vi "InsertReportSection.vi"(8 "error in (no error)":errorcluster, 10 "report entry":string, 11 "report section in":refnum<k7>) -> (0 "error out":errorcluster, 3 "report section out":refnum<k7>)   [LabVIEW 2019]
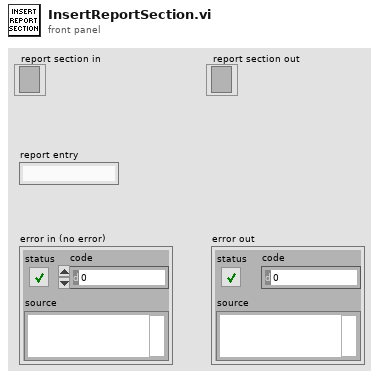
[diagram p1: front panel]
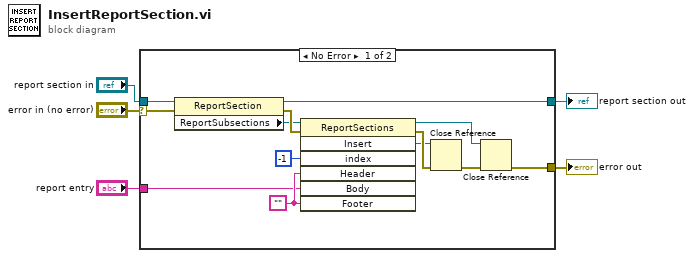
[diagram p0: block diagram]
diagram:
  n1 = case shown="No Error" "error in (no error)" {
    selector: "error in (no error)" -> [w6 w19]
    tunnel: [w16 w19] -> w5
    tunnel: "report entry" -> [w10 _]
    tunnel: [w8 w20] -> w3
    tunnel: "report section in" -> [w7 w20]
    frame No Error {
      w12 = ""
      n2 = property class="ReportSection"(reference=w7, error in=w6) -> (reference out=w8:refnum<k7>, error out=w18:errorcluster, "ReportSubsections"=w9:refnum<k7>)
      n3 = invoke class="ReportSections" method="Insert"(reference=w9, error in=w18, "index"=-1, "Header"=w12, "Body"=w10, "Footer"=w12) -> (reference out=w14:refnum<k7>, error out=w17:errorcluster, "Insert"=w13:refnum<k7>)  [unwired: 1 in, 4 out]
      n4 = Close Reference(reference=w13, error in (no error)=w17) -> (error out=w15:errorcluster)
      n5 = Close Reference(reference=w14, error in (no error)=w15) -> (error out=w16:errorcluster)
    }
    frame Error {
    }
  }
  "error out" <- w5
  "report section out" <- w3
